vi "CIPC Channel Errors.vi"(8 "error in (no error)":errorcluster, 9 "String to Append":string, 10 "Error":T1, 11 "Insert Error":bool=TRUE) -> (0 "error out":errorcluster)   [LabVIEW 2021, in "CIF_CIPC_Chn.lvclass"]
uses:
  CIF_CIPC_Chn.lvclass
  Typedef/CIPC Channel Error.ctl
  CIF_CIPC_Chn.lvclass/CIF_CIPC_Chn.ctl
  <vilib>/CIF Foundation/CIF Utilities/Errors/Errors_CIF_U.lvlib
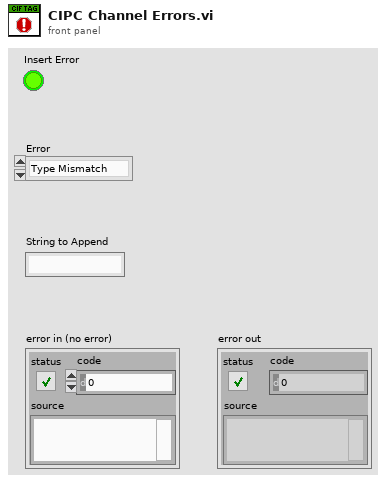
[diagram p1: front panel]
types:
  T1 = typedef "CIF_CIPC_Chn.lvclass/CIPC Channel Error.ctl" = enum16{"Type Mismatch"}
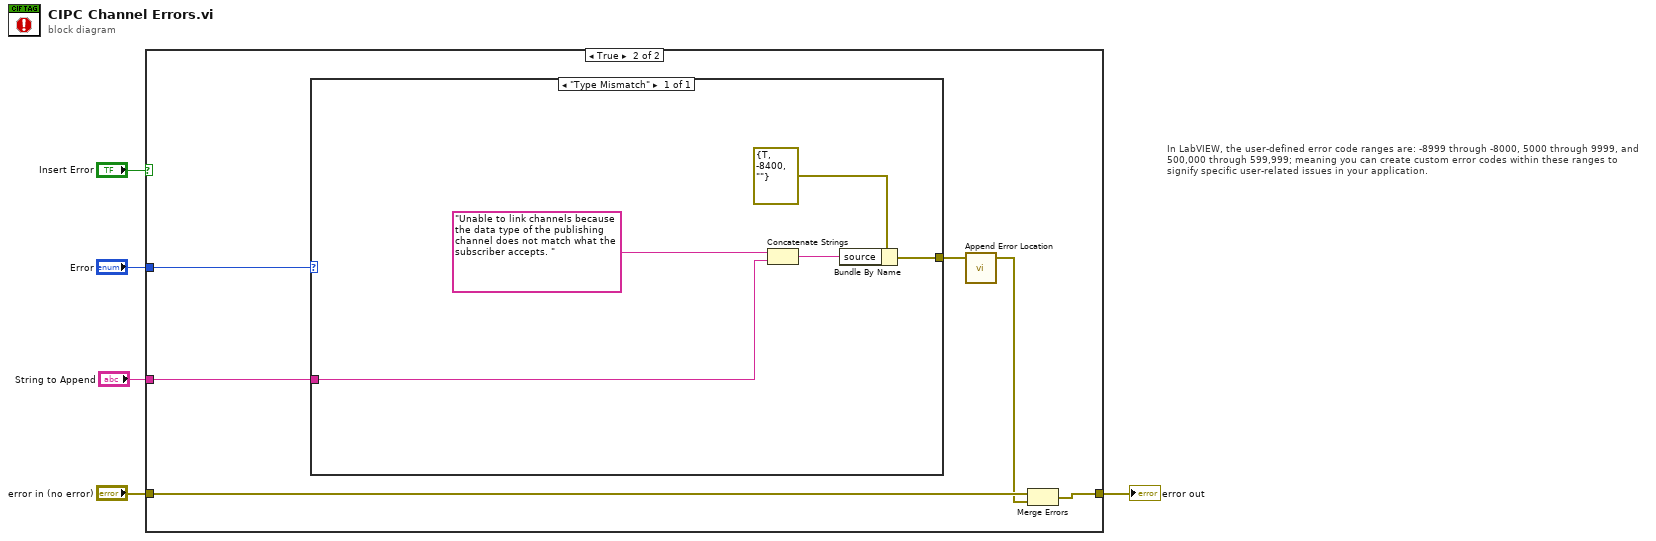
[diagram p0: block diagram]
diagram:
  # "In LabVIEW, the user-defined error code ranges are: -8999 through -8000, 5000 through 9999, and 500,000 through 599,999; meaning you can create custom error codes within these ranges to signify specific user-related issues in your application."
  n1 = case shown="True" "Insert Error" {
    tunnel: [w6 w9] -> w4
    tunnel: "error in (no error)" -> [w6 w10]
    tunnel: "Error" -> [_ w12]
    tunnel: "String to Append" -> [_ w11]
    frame False {
    }
    frame True {
      n2 = case shown="\"Type Mismatch\"" w12 {
        tunnel: w11 -> [w13]
        tunnel: [w16] -> w8
        frame "Type Mismatch" {
          n3 = Concatenate Strings("Unable to link channels because the data type of the publishing channel does not match what the subscriber accepts. " ("source"), w13) -> (w14:string)
          n4 = Bundle By Name(cluster=errorcluster {"status"=TRUE, "code"=-8400, "source"=""} ("Invalid ID"), "source"=w14) -> (w16:errorcluster)
        }
      }
      n5 = call <vilib>:"Append Error Location.vi"("error in (no error)"=w8) -> ("error out"=w7:errorcluster)  [unwired: 4 in]
      n6 = Merge Errors(w10, w7) -> (w9:errorcluster)
    }
  }
  "error out" <- w4
